vi "MOCK_FP_Read_Boolean.vi"(7 "Type":bool=TRUE, 8 "error in":errorcluster, 11 "FieldPoint IO Point In":refnum<k21>) -> (0 "error out":errorcluster, 1 "timestamp":dbl format="%.2f", 2 "Boolean":bool=TRUE, 3 "FieldPoint IO Point Out":refnum<k21>)   [LabVIEW 2017]
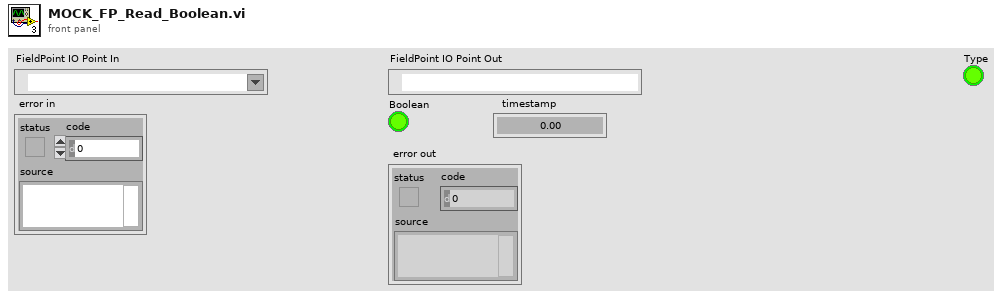
[diagram p1: front panel]
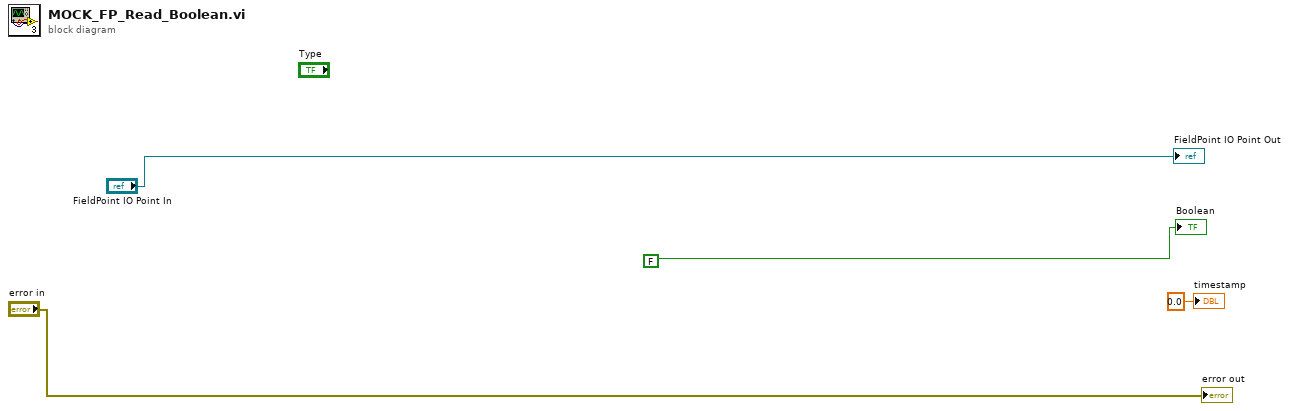
[diagram p0: block diagram]
diagram:
  "FieldPoint IO Point Out" <- "FieldPoint IO Point In"
  "timestamp" <- 0.0 ("timestamp")
  "error out" <- "error in"
  "Boolean" <- FALSE
